vi "StopServer.vi"(8 "error in (no error)":errorcluster) -> (0 "error out":errorcluster)   [LabVIEW 2010, in "MonitorServer.lvlib"]
uses:
  MonitorServer.lvlib
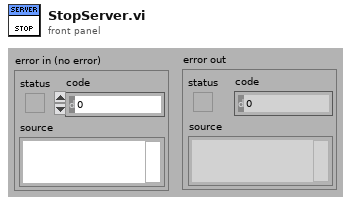
[diagram p1: front panel]
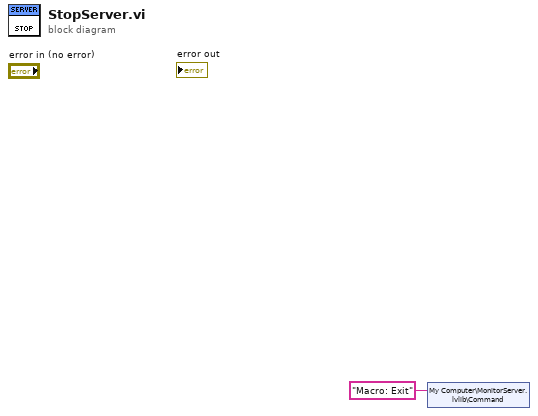
[diagram p0: block diagram]
diagram:
  n1 = shared-variable "My Computer\\MonitorServer.lvlib\\Command"("Macro: Exit" ("Command")) -> ()  [unwired: 1 in, 1 out]
